vi "SubPanel_Cord In Range.vi"(7 "Coords":T1, 8 "Top":i32, 9 "Height":u32, 10 "Left":i32, 11 "Width":u32) -> (3 "In Range Out":bool)   [LabVIEW 2020]
uses:
  <vilib>/Utility/miscctls.llb/LVPoint32TypeDef.ctl
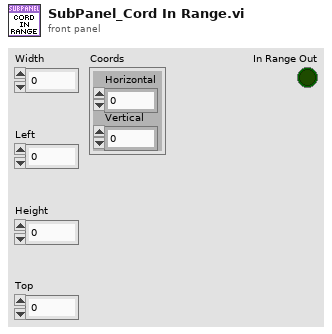
[diagram p1: front panel]
types:
  T1 = typedef "LVPoint32TypeDef.ctl" = cluster{"Horizontal":i32, "Vertical":i32}
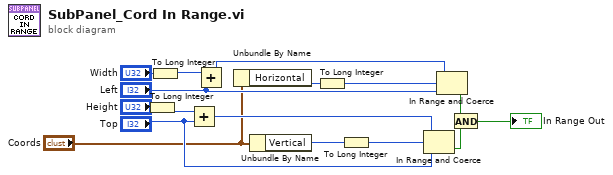
[diagram p0: block diagram]
diagram:
  n1 = To Long Integer(number="Height") -> (32bit integer=w3:i32)
  n2 = To Long Integer(number="Width") -> (32bit integer=w4:i32)
  n3 = Add(x=w3, y="Top") -> (x+y=w11:i32)
  n4 = Add(x=w4, y="Left") -> (x+y=w13:i32)
  n5 = Unbundle By Name("Coords") -> ("Horizontal"=w7:i32)
  n6 = Unbundle By Name("Coords") -> ("Vertical"=w5:i32)
  n7 = To Long Integer(number=w7) -> (32bit integer=w2:i32)
  n8 = To Long Integer(number=w5) -> (32bit integer=w1:i32)
  n9 = In Range and Coerce(upper limit=w11, x=w1, lower limit="Top") -> (In Range?=w9:bool)  [unwired: 1 out]
  n10 = In Range and Coerce(upper limit=w13, x=w2, lower limit="Left") -> (In Range?=w10:bool)  [unwired: 1 out]
  n11 = And(x=w10, y=w9) -> (x .and. y?=→"In Range Out":bool)
